vi "Safe vs Unsafe.vi"(5 "Show Cache Lines (F)":bool, 7 "Show Peak Bandwidth (F)":bool, 9 "Transfers (500)":i32=500, 10 "End Size":u64=50000000 format="%.0pB", 11 "Start Size":u64=1000 format="%.0pB") -> ()   [LabVIEW 2016]
panel:
  out "Peak Throughput (Safe)":dbl format="%.3pB/s"
  out "Peak Throughput (Unsafe)":dbl format="%.3pB/s"
  out "Memory Bandwidth (Safe)":cluster{"X":dbl[], "Y":dbl[]}[](graph) caption="Memory Bandwidth Plot"
  out "Memory Bandwidth (Unsafe)":cluster{"X":dbl[], "Y":dbl[]}[](graph) caption="Memory Bandwidth Plot"
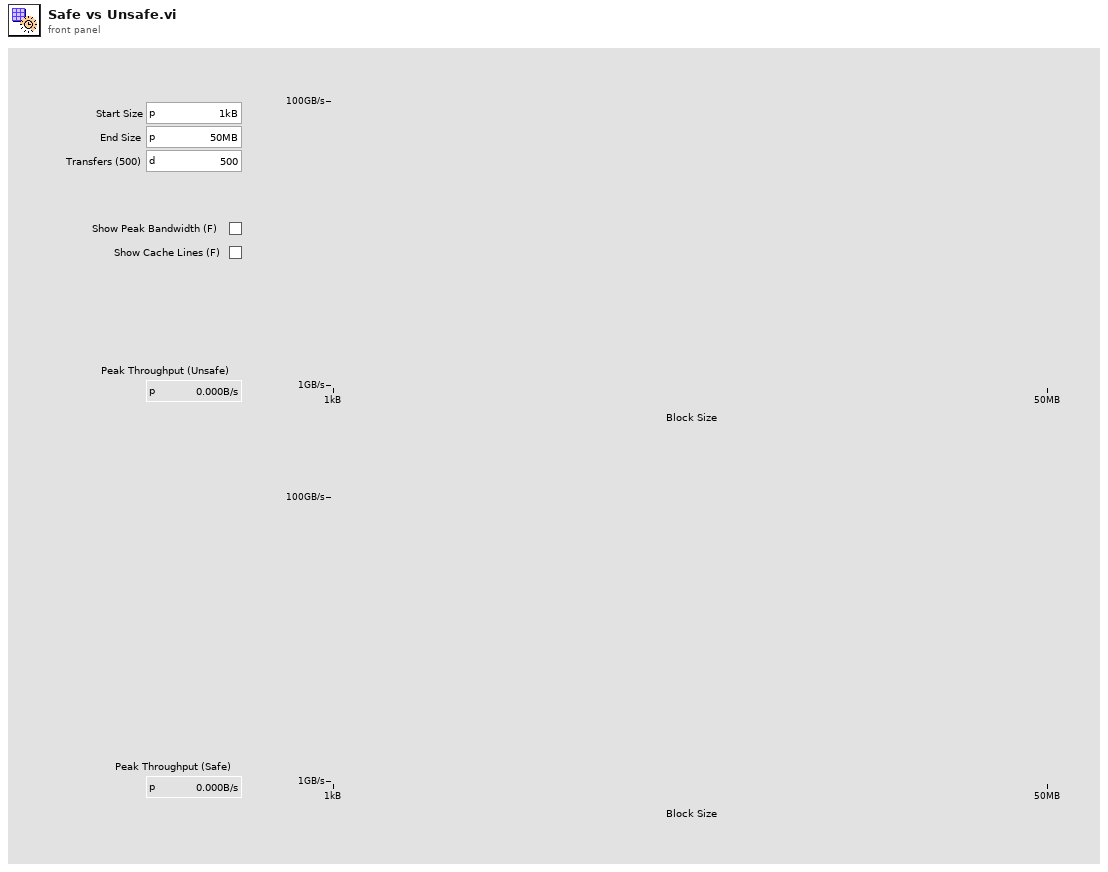
[diagram p1: front panel]
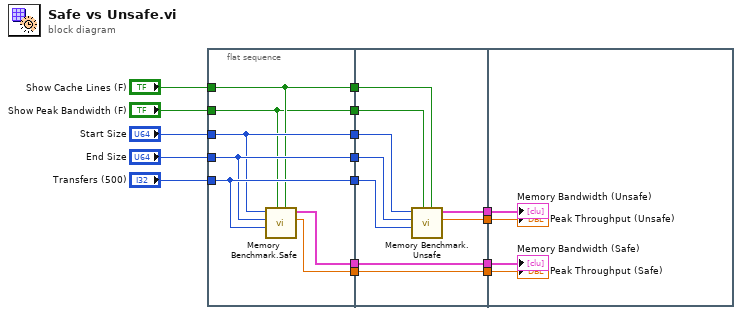
[diagram p0: block diagram]
diagram:
  n1 = flat-sequence {
    tunnel: "End Size" -> [w22]
    tunnel: "Start Size" -> [w21]
    tunnel: "Show Peak Bandwidth (F)" -> [w19]
    tunnel: "Show Cache Lines (F)" -> [w20]
    tunnel: "Transfers (500)" -> [w23]
    tunnel: [w23] -> w11
    tunnel: [w22] -> w10
    tunnel: [w21] -> w9
    tunnel: [w20] -> w8
    tunnel: [w19] -> w7
    tunnel: [w18] -> w6
    tunnel: [w17] -> w2
    tunnel: w11 -> [w32]
    tunnel: w10 -> [w31]
    tunnel: w9 -> [w30]
    tunnel: w8 -> [w28]
    tunnel: w7 -> [w29]
    tunnel: w6 -> [w27]
    tunnel: [w27] -> w5
    tunnel: [w26] -> w4
    tunnel: [w25] -> w3
    tunnel: w2 -> [w24]
    tunnel: [w24] -> w1
    tunnel: w5 -> [w35]
    tunnel: w4 -> [w36]
    tunnel: w3 -> [w33]
    tunnel: w1 -> [w34]
    frame #0 {
      n2 = call "Memory Benchmark.Safe.vi"("Show Cache Lines (F)"=w20, "Show Peak Bandwidth (F)"=w19, "Transfers (500)"=w23, "End Size"=w22, "Start Size"=w21) -> ("Peak Throughput"=w17:dbl, "Memory Bandwidth"=w18:cluster{"X":dbl[], "Y":dbl[]}[])  [unwired: 5 in]
    }
    frame #1 {
      n3 = call "Memory Benchmark.Unsafe.vi"("Show Cache Lines (F)"=w28, "Show Peak Bandwidth (F)"=w29, "Transfers (500)"=w32, "End Size"=w31, "Start Size"=w30) -> ("Peak Throughput"=w25:dbl, "Memory Bandwidth"=w26:cluster{"X":dbl[], "Y":dbl[]}[])  [unwired: 5 in]
    }
    frame #2 {
      "Memory Bandwidth (Safe)" <- w35
      "Memory Bandwidth (Unsafe)" <- w36
      "Peak Throughput (Unsafe)" <- w33
      "Peak Throughput (Safe)" <- w34
    }
  }
